vi "pfeil_in_abhänigkeit_der_fahrtrichtung_drehen.vi"(10 "Angle in":sgl, 11 "Array":dbl[][](array[numeric])) -> (3 "Angle out":sgl)   [LabVIEW 2014]
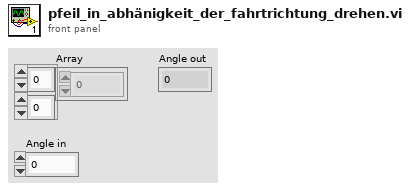
[diagram p1: front panel]
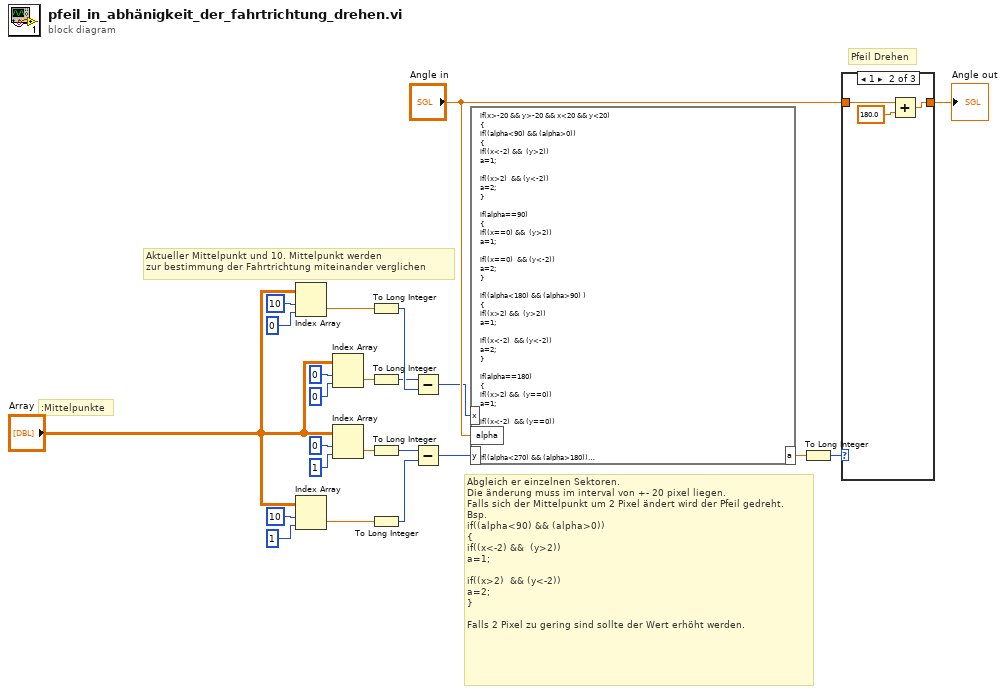
[diagram p0: block diagram]
diagram:
  # "Pfeil Drehen"
  # "Aktueller Mittelpunkt und 10. Mittelpunkt werden \nzur bestimmung der Fahrtrichtung miteinander verglichen"
  # ":Mittelpunkte"
  # "Abgleich er einzelnen Sektoren.\nDie änderung muss im interval von +- 20 pixel liegen.\nFalls sich der Mittelpunkt um 2 Pixel ändert wird der Pfeil gedreht.\nBsp. \nif((alpha<90) && (alpha>0))\n{\nif((x<-2) &&  (y>2))\na=1;\n\nif((x>2)  && (y<-2))\na=2;\n} \n\nFalls 2 Pixel zu gering sind sollte der Wert erhöht werden."
  n1 = Index Array(array="Array", index (row)=10, index (col)=0) -> (element=w12:dbl)
  n2 = Index Array(array="Array", index (row)=10, index (col)=1) -> (element=w11:dbl)
  n3 = Index Array(array="Array", index (row)=0, index (col)=0) -> (element=w10:dbl)
  n4 = Index Array(array="Array", index (row)=0, index (col)=1) -> (element=w9:dbl)
  n5 = To Long Integer(number=w12) -> (32bit integer=w14:i32)
  n6 = To Long Integer(number=w10) -> (32bit integer=w13:i32)
  n7 = To Long Integer(number=w9) -> (32bit integer=w15:i32)
  n8 = To Long Integer(number=w11) -> (32bit integer=w16:i32)
  n9 = Subtract(x=w13, y=w14) -> (x-y=w20:i32)
  n10 = Subtract(x=w15, y=w16) -> (x-y=w22:i32)
  n11 = formula code="if(x>-20 && y>-20 && x<20 && y<20)\n{\nif((alpha<90) && (alpha>0))\n{\nif((x<-2) &&  (y>2))\na=1;\n\nif((x>2)  && (y<-2))\na=2;\n}\n\nif(alpha==90)\n{\nif((x==0) &&  (y>2))\na=1;\n\nif((x==0)  && (y<-2))\na=2;\n}\n\nif((alpha<180) && (alpha>90) )\n{\nif((x>2) &&  (y>2))\na=1;\n\nif((x<-2)  && (y<-2))\na=2;\n}\n\nif(alpha==180)\n{\nif((x>2) &&  (y==0))\na=1;\n\nif((x<-2)  && (y==0))\na=2;\n}\n\nif((alpha<270) && (alpha>180))\n{\nif((x>2) &&  (y<-2))\na=1;\n\nif((x<-2)  && (y>2))\na=2;\n}\n\nif(alpha==270)\n{\nif((x>2) &&  (y==0))\na=1;\n\nif((x<-2)  && (y==0))\na=2;\n}\n\n\nif((alpha<360) && (alpha>270))\n{\nif((x<-2) &&  (y<-2))\na=1;\n\nif((x>2)  && (y>2))\na=2;\n}\n}"("x"=w20, "y"=w22, "alpha"="Angle in") -> ("a"=w23:dbl)
  n12 = To Long Integer(number=w23) -> (32bit integer=w17:i32)
  n13 = case shown="1" w17 {
    tunnel: "Angle in" -> [w24 w27 w28]
    tunnel: [w24 w26 w28] -> w19
    frame 0, Default {
    }
    frame 1 {
      n14 = Add(x=w27, y=sgl 180.0) -> (x+y=w26:sgl)
    }
    frame 2 {
    }
  }
  "Angle out" <- w19
